vi "FPGA_PPG_application_example.vi"() -> ()   [LabVIEW 2014, in "NI-FPGA_PPG_Driver.lvlib"]
doc: "A simple application example for producing a few bit patterns with the FPGA.\n\nDietrich Beck, GSI Helmholtzzentrum fuer Schwerionenforschung, Germany"
uses:
  NI-FPGA_PPG_Driver.lvlib
  target/FPGA_target_state_type.ctl
panel:
  in  "Load?":bool
  in  "save?":bool
  in  "mode":u8(ring) items=["once", "continous"]
  in  "stop":bool
  in  "command_lines 2":string[](array[string])=["$time::1::1::0", "$time::9::0::0", "$time::0.05::2::0", "$time::0.45::0::0", "$time::0.05::6::0", "$time::0.45::0::0", "$time::0.05::14::0", "$time::0.45::0::0", "$time::0.05::2::0", "$time::10000::0::0"]
  out "FPGA_state":T1
  in  "waitOnTrigger":bool
  out "Numeric":i32
  out "error out":errorcluster
  in  "resource_in":refnum<visa-resource-name>="RIO0::INSTR"
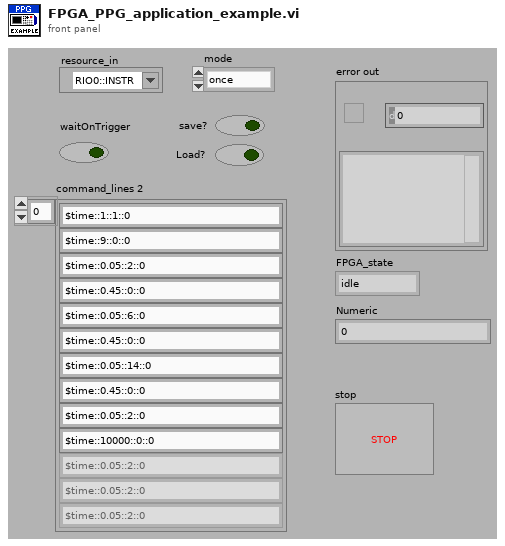
[diagram p1: front panel]
types:
  T1 = typedef "NI-FPGA_PPG_Driver.lvlib/FPGA_target_state_type.ctl" = enum16{"idle", "reset", "query", "load", "run", "stopped"}
  T2 = enum8{"Enabled", "Disabled", "Disabled and Grayed Out"}
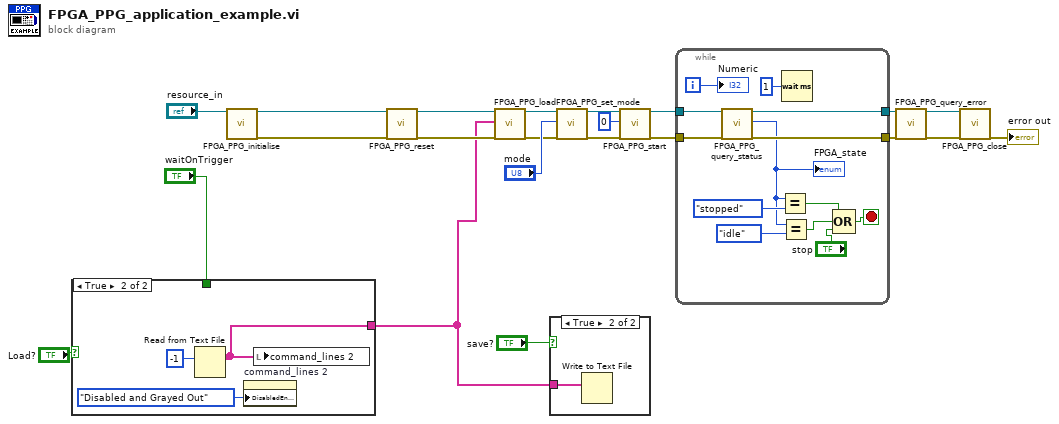
[diagram p0: block diagram]
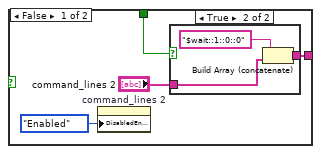
[diagram p2: hidden frame]
diagram:
  n1 = case shown="True" "Load?" {
    tunnel: "waitOnTrigger" -> [w24 _]
    tunnel: [w23 w31] -> w1
    frame False {
      n2 = property on="command_lines 2" class="Arr (strict)"("DisabledEnum"=T2."Enabled" ("Disabled")) -> ()  [unwired: 2 in, 2 out]
      n3 = case shown="True" w24 {
        tunnel: "command_lines 2" -> [w27 w29]
        tunnel: [w27 w28] -> w23
        frame False {
        }
        frame True {
          n4 = Build Array (concatenate)("$wait::1::0::0", w29) -> (w28:string[])
        }
      }
    }
    frame True {
      n5 = Read from Text File(count=-1) -> (text=w31:string[])  [unwired: 3 in, 3 out]
      n6 = property on="command_lines 2" class="Arr (strict)"("DisabledEnum"=T2."Disabled and Grayed Out" ("Disabled")) -> ()  [unwired: 2 in, 2 out]
      n7 = local write "command_lines 2"(w31) -> ()
    }
  }
  n8 = call "FPGA_PPG_initialise.vi"("resource_in"="resource_in") -> ("resource_out"=w8:refnum<visa-resource-name>, "error out"=w6:errorcluster)  [unwired: 16 in, 1 out]
  n9 = call "FPGA_PPG_reset.vi"("resource_in"=w8, "error in (no error)"=w6) -> ("resource_out"=w7:refnum<visa-resource-name>, "error out"=w5:errorcluster)  [unwired: 16 in]
  n10 = call "FPGA_PPG_load.vi"("resource_in"=w7, "command_lines"=w1, "error in (no error)"=w5) -> ("resource_out"=w9:refnum<visa-resource-name>, "error out"=w10:errorcluster)  [unwired: 15 in]
  n11 = case shown="True" "save?" {
    tunnel: w1 -> [_ w34]
    frame False {
    }
    frame True {
      n12 = Write to Text File(text=w34) -> ()  [unwired: 3 in, 3 out]
    }
  }
  n13 = call "FPGA_PPG_set_mode.vi"("resource_in"=w9, "mode"="mode", "error in (no error)"=w10) -> ("resource_out"=w13:refnum<visa-resource-name>, "error out"=w12:errorcluster)  [unwired: 15 in]
  n14 = call "FPGA_PPG_start.vi"("resource_in"=w13, "start_addr"=u32 0, "error in (no error)"=w12) -> ("resource_out"=w21:refnum<visa-resource-name>, "error out"=w20:errorcluster)  [unwired: 15 in]
  n15 = while {
    tunnel: w21 -> [w47]
    tunnel: w20 -> [w46]
    tunnel: [w45] -> w18
    tunnel: [w44] -> w17
    i -> [w43]
    stop <- w36 stop-if-true
    n16 = call "FPGA_PPG_query_status.vi"("resource_in"=w47, "error in (no error)"=w46) -> ("resource_out"=w44:refnum<visa-resource-name>, "FPGA_state"=w40:T1, "error out"=w45:errorcluster)  [unwired: 15 in]
    "FPGA_state" <- w40
    n17 = Equal?(x=w40, y=FPGA_target_state_type."stopped") -> (x = y?=w37:bool)
    n18 = Equal?(x=w40, y=FPGA_target_state_type."idle") -> (x = y?=w38:bool)
    n19 = Wait (ms)(milliseconds to wait=u32 1) -> ()  [unwired: 1 out]
    n20 = Compound Arithmetic op=OR(w37, w38, "stop") -> (w36:bool)
    "Numeric" <- w43
  }
  n21 = call "FPGA_PPG_query_error.vi"("resource_in"=w17, "error in (no error)"=w18) -> ("resource_out"=w15:refnum<visa-resource-name>, "error out"=w16:errorcluster)  [unwired: 16 in]
  n22 = call "FPGA_PPG_close.vi"("resource_in"=w15, "error in (no error)"=w16) -> ("error out"=→"error out":errorcluster)  [unwired: 17 in]
